vi "Interface.RT FIFO.Read.vi"   [LabVIEW 2017, in "DSF Core.lvlib" / "Interface.lvclass"]
uses:
  Interface.lvclass
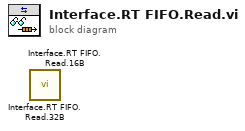
[diagram p0: block diagram]
diagram:
  n1 = call "Interface.RT FIFO.Read.32B.vi"() -> ()  [unwired: 7 in, 5 out]
  n2 = call "Interface.RT FIFO.Read.16B.vi"() -> ()  [unwired: 7 in, 5 out]
